vi "Get Tag from Enqueuer.vi"(10 "Enqueuer":refnum<class "Message Enqueuer.lvclass">=refnum) -> (2 "Tag":string)   [LabVIEW 2023, in "Monitored Actor.lvlib" / "Classic Monitor.lvclass"]
doc: "Converts the enqueuer object to a tree-compatible tag\n\nCopyright: MGI 2016\nAuthor: Derek Trepanier"
uses:
  Classic Monitor.lvclass
  builds/Framework/Actor Framework.lvlibp/1abvi3w/vi.lib/ActorFramework/Message Enqueuer/Message Enqueuer.lvclass
  Classic Monitor.lvclass/Classic Monitor.ctl
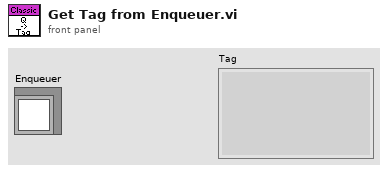
[diagram p1: front panel]
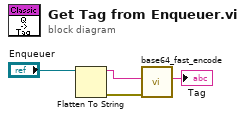
[diagram p0: block diagram]
diagram:
  n1 = Flatten To String(anything="Enqueuer") -> (data string=w3:string, error out=w2:errorcluster)  [unwired: 3 in, 1 out]
  n2 = call "base64_fast_encode.vi"("error in (no error)"=w2, "string in (not encoded)"=w3) -> ("string out (base64-encoded)"=→"Tag":string)  [unwired: 8 in, 1 out]
